vi "Teleop_old_317.vi"(10 "Match Info":T1={"Autonomous Elapsed Seconds"=0.0, "TeleOp Elapsed Seconds"=0.0, "Disabled Elapsed Seconds"=0.0, "Visited Autonomous"=FALSE, "Visited TeleOp"=FALSE, "Visited Disabled"=FALSE, "Autonomous Settings"={"Autonomous Style"=enum."Independent", "VI Refnum"=refnum}}, 11 "Call Context":T2) -> ()   [LabVIEW 2016]
doc: "This VI is called for each TeleOp packet received from the DS where the robot is not disabled. It is often used to read from the joysticks and update I/O or to update setpoints for timed control loops. It should complete and return within 20 milliseconds or it may miss DS packets."
uses:
  <vilib>/Rock Robotics/WPI/DriverStation/WPI_DriverStationDerivedRobotMode.ctl
  <vilib>/Rock Robotics/WPI/DriverStation/WPI_DriverStationMatch Info.ctl
  <vilib>/Rock Robotics/WPI/Relay/WPI_RelayValue.ctl
  <vilib>/Rock Robotics/WPI/Solenoid/WPI_SolenoidValue.ctl
  <vilib>/Rock Robotics/WPI/Utilities/WPI_GetSetVariantRefNum.vi
  <vilib>/Rock Robotics/Network Tables/NT Write Boolean Array.vi
  <vilib>/Rock Robotics/Network Tables/NT Write Numeric Array.vi
  <vilib>/Rock Robotics/Network Tables/NT Read Boolean.vi
  <vilib>/Rock Robotics/Network Tables/NT Read Number.vi
  <vilib>/Rock Robotics/WPI/Solenoid/WPI_SolenoidSetEnum.vi
panel:
  out "Feed 2":dbl(slide) scale=-1.0..1.0
  out "Feed":dbl(slide) scale=-1.0..1.0
  out "Sample Slider 0":dbl(slide) scale=0.0..5.0
  out "Sample Boolean 1":bool
  out "Sample Boolean 0":bool
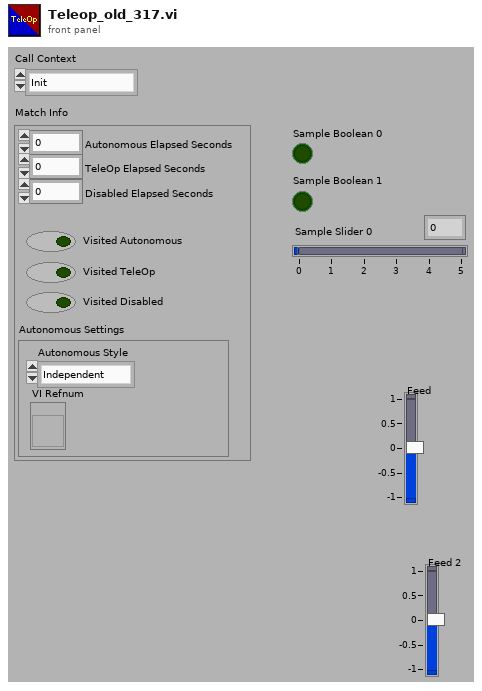
[diagram p1: front panel]
types:
  T1 = typedef "WPI_DriverStationMatch Info.ctl" = cluster{"Autonomous Elapsed Seconds":dbl, "TeleOp Elapsed Seconds":dbl, "Disabled Elapsed Seconds":dbl, "Visited Autonomous":bool, "Visited TeleOp":bool, "Visited Disabled":bool, "Autonomous Settings":cluster{"Autonomous Style":enum16{"Iterative", "Independent"}, "VI Refnum":refnum<vi>}}
  T2 = typedef "WPI_DriverStationDerivedRobotMode.ctl" = enum16{"Init", "Execute", "Stop"}
  T3 = typedef "WPI_JoystickDevRef.ctl" = cluster{"Device":T4}
  T4 = typedef "WPI_JoystickDeviceEnum.ctl" = enum16{"USB 0", "USB 1", "USB 2", "USB 3", "USB 4", "USB 5"}
  T5 = cluster{"Buttons[0]":bool, "Buttons[1]":bool, "Buttons[2]":bool, "Buttons[3]":bool, "Buttons[4]":bool, "Buttons[5]":bool, "Buttons[6]":bool, "Buttons[7]":bool, "Buttons[8]":bool, "Buttons[9]":bool, "Buttons[10]":bool}
  T6 = typedef "WPI_MotorControlDeviceRef.ctl" = cluster{"DeviceStatus":errorcluster, "Type":T7, "PWM":cluster{"PWM Channel":T8, "DeadBand":T9}, "CAN":cluster{"Device Number":u8, "SetOutput VI Ref":variant, "GetOutput VI Ref":variant, "Enable VI Ref":variant, "Disable VI Ref":variant, "Data":variant}, "Invert":bool}
  T7 = typedef "WPI_MotorControlType.ctl" = enum16{"PWM", "CAN"}
  T8 = typedef "FPGA_DIOPWMChannel.ctl" = enum8{"PWM 0", "PWM 1", "PWM 2", "PWM 3", "PWM 4", "PWM 5", "PWM 6", "PWM 7", "PWM 8", "PWM 9", "PWM MXP 0", "PWM MXP 1", "PWM MXP 2", "PWM MXP 3", "PWM MXP 4", "PWM MXP 5", "PWM MXP 6", "PWM MXP 7", "PWM MXP 8", "PWM MXP 9", "Invalid"}
  T9 = typedef "WPI_PWMDeadband.ctl" = cluster{"Name":string, "maxPositivePwm":i32, "minPositivePwm":i32, "centerPwm":i32, "maxNegativePwm":i32, "minNegativePwm":i32, "angularRange":u16}
  T10 = typedef "WPI_RelayDevRef.ctl" = cluster{"DevStatus":errorcluster, "Relay Channel":T11, "Relay Direction":T12}
  T11 = typedef "FPGA_DIORelayChannel.ctl" = enum8{"Relay 0", "Relay 1", "Relay 2", "Relay 3", "Invalid"}
  T12 = typedef "WPI_RelayDirection.ctl" = enum16{"Both directions", "Forward only", "Reverse only"}
  T13 = typedef "WPI_RobotDriveDevRef.ctl" = cluster{"DevStatus":errorcluster, "Motors[]":T6[], "Square Inputs":bool, "Max Output":dbl}
  T14 = typedef "WPI_SolenoidDevRef.ctl" = cluster{"DevStatus":errorcluster, "Pneumatics Control Module":u8, "Forward Solenoid Channel":T15, "Reverse Solenoid Channel":T15}
  T15 = typedef "WPI_SolenoidChannel.ctl" = enum8{"Solenoid 0", "Solenoid 1", "Solenoid 2", "Solenoid 3", "Solenoid 4", "Solenoid 5", "Solenoid 6", "Solenoid 7", "Invalid"}
  T16 = cluster{"Axes[0]":dbl, "Axes[1]":dbl, "Axes[2]":dbl, "Axes[3]":dbl, "Axes[4]":dbl, "Axes[5]":dbl, "Axes[6]":dbl, "Axes[7]":dbl, "Axes[8]":dbl}
  T17 = typedef "WPI_SolenoidValue.ctl" = enum16{"Off", "On", "Forward", "Reverse"}
  T18 = typedef "WPI_RelayValue.ctl" = enum16{"Off", "On", "Forward", "Reverse"}
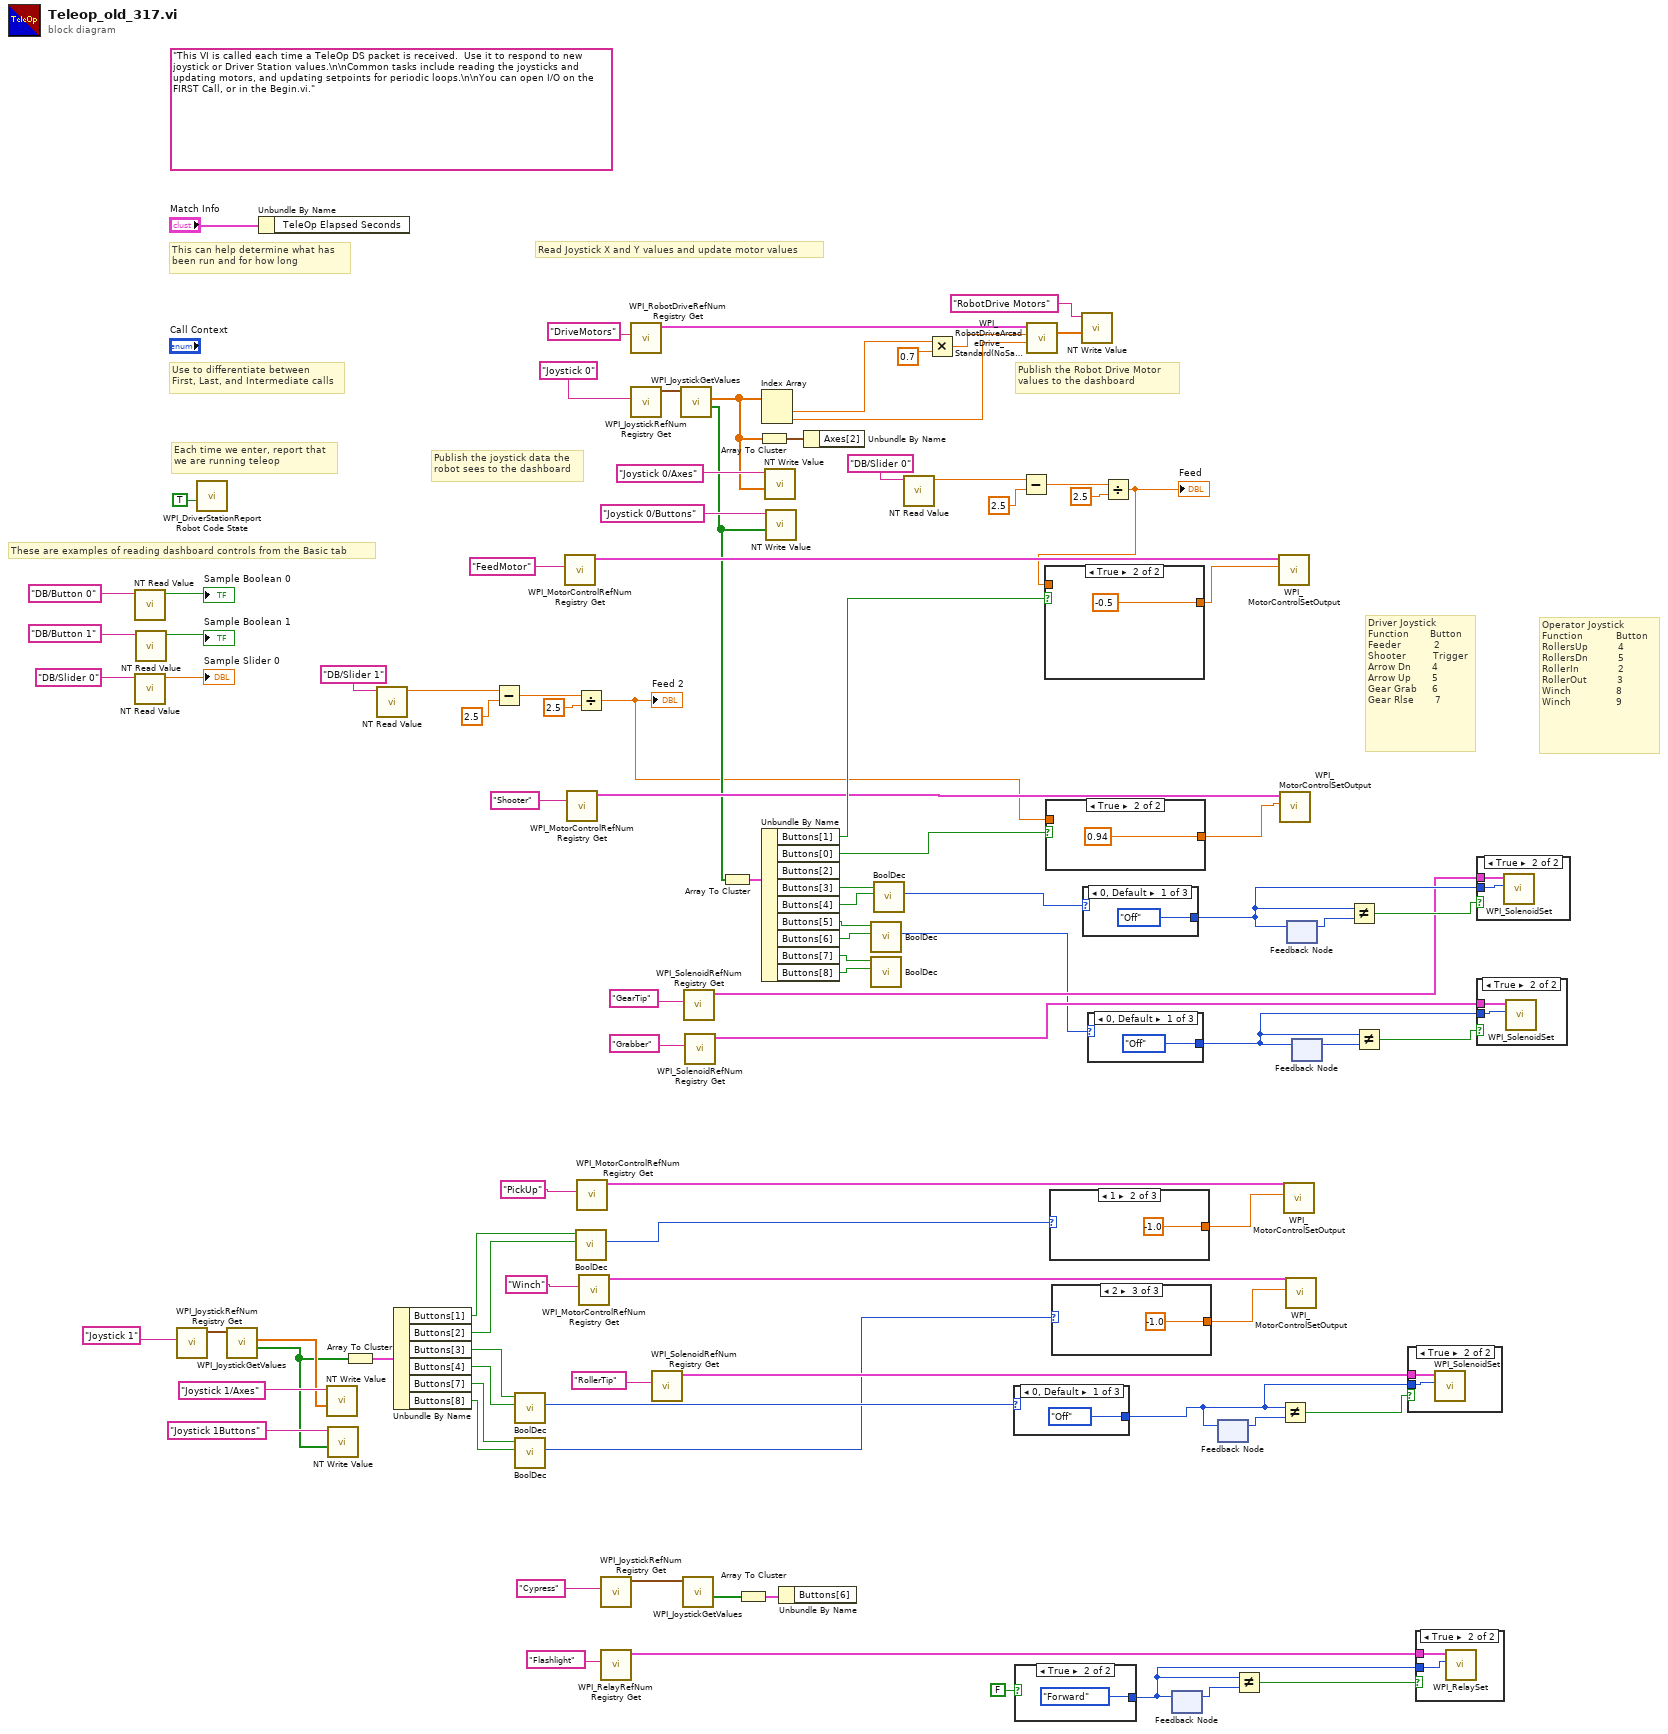
[diagram p0: block diagram]
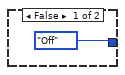
[diagram p3: hidden frame]
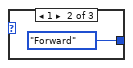
[diagram p4: hidden frame]
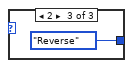
[diagram p5: hidden frame]
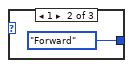
[diagram p6: hidden frame]
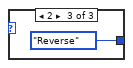
[diagram p7: hidden frame]
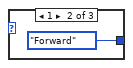
[diagram p11: hidden frame]
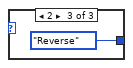
[diagram p12: hidden frame]
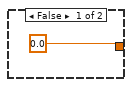
[diagram p13: hidden frame]
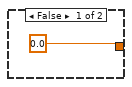
[diagram p14: hidden frame]
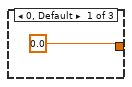
[diagram p15: hidden frame]
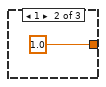
[diagram p16: hidden frame]
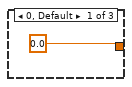
[diagram p17: hidden frame]
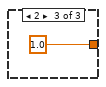
[diagram p18: hidden frame]
diagram:
  (unwired) "This VI is called each time a TeleOp DS packet is received.  Use it to respond to new joystick or Driver Station values.\n\nCommon tasks include reading the joysticks and updating motors, and updating setpoints for periodic loops.\n\nYou can open I/O on the FIRST Call, or in the Begin.vi."
  # "Operator Joystick\nFunction           Button\nRollersUp          4\nRollersDn          5\nRollerIn             2\nRollerOut          3\nWinch               8\nWinch               9"
  # "Driver Joystick\nFunction       Button\nFeeder           2\nShooter         Trigger\nArrow Dn       4\nArrow Up       5\nGear Grab     6\nGear Rlse       7"
  # "These are examples of reading dashboard controls from the Basic tab"
  # "Publish the Robot Drive Motor\nvalues to the dashboard"
  # "Publish the joystick data the\nrobot sees to the dashboard"
  # "Each time we enter, report that\nwe are running teleop"
  # "Use to differentiate between\nFirst, Last, and Intermediate calls"
  # "This can help determine what has\nbeen run and for how long"
  # "Read Joystick X and Y values and update motor values"
  n1 = call-poly <vilib>:"NT Read Value.vi"("Name"="DB/Button 0" ("refnum name")) -> ("Boolean"=→"Sample Boolean 0":bool)  [unwired: 9 in, 1 out]
  n2 = call-poly <vilib>:"NT Read Value.vi"("Name"="DB/Slider 0" ("refnum name")) -> ("Numeric"=→"Sample Slider 0":dbl)  [unwired: 9 in, 1 out]
  n3 = call-poly <vilib>:"NT Read Value.vi"("Name"="DB/Button 1" ("refnum name")) -> ("Boolean"=→"Sample Boolean 1":bool)  [unwired: 9 in, 1 out]
  n4 = call <vilib>:"WPI_JoystickRefNum Registry Get.vi"("refnum name"="Joystick 1") -> ("JoystickDevRef"=w63:T3)  [unwired: 1 in, 9 out]
  n5 = call <vilib>:"WPI_DriverStationReport Robot Code State.vi"("TeleOp"=TRUE ("Autonomous")) -> ()  [unwired: 10 in, 1 out]
  n6 = call <vilib>:"WPI_JoystickGetValues.vi"("JoystickDevRef"=w63) -> ("Buttons"=w53:bool[], "Axes"=w59:dbl[])  [unwired: 6 in, 3 out]
  n7 = Unbundle By Name("Match Info") -> ()  [unwired: 1 out]
  n8 = call-poly <vilib>:"NT Write Value.vi"("Numeric Array"=w59, "Name"="Joystick 1/Axes") -> ()  [unwired: 9 in, 1 out]
  n9 = call-poly <vilib>:"NT Write Value.vi"("Boolean Array"=w53, "Name"="Joystick 1Buttons") -> ()  [unwired: 9 in, 1 out]
  n10 = Array To Cluster(array=w53) -> (cluster=w52:T5)
  n11 = call-poly <vilib>:"NT Read Value.vi"("Name"="DB/Slider 1") -> ("Numeric"=w24:dbl)  [unwired: 9 in, 1 out]
  n12 = Unbundle By Name(w52) -> ("Buttons[1]"=w49:bool, "Buttons[2]"=w48:bool, "Buttons[3]"=w51:bool, "Buttons[4]"=w50:bool, "Buttons[7]"=w43:bool, "Buttons[8]"=w42:bool)
  n13 = Subtract(x=w24, y=2.5) -> (x-y=w22:dbl)
  n14 = call "BoolDec.vi"("Bit0"=w51, "Bit1"=w50) -> ("Out"=w7:i8)  [unwired: 8 in]
  n15 = call "BoolDec.vi"("Bit0"=w43, "Bit1"=w42) -> ("Out"=w5:i8)  [unwired: 8 in]
  n16 = call <vilib>:"WPI_MotorControlRefNum Registry Get.vi"("refnum name"="FeedMotor") -> ("MotorControlDevRef"=w66:T6)  [unwired: 9 in, 1 out]
  n17 = call <vilib>:"WPI_MotorControlRefNum Registry Get.vi"("refnum name"="Shooter") -> ("MotorControlDevRef"=w67:T6)  [unwired: 9 in, 1 out]
  n18 = Divide(x=w22, y=2.5) -> (x/y=w14:dbl)
  "Feed 2" <- w14
  n19 = call "BoolDec.vi"("Bit0"=w49, "Bit1"=w48) -> ("Out"=w6:i8)  [unwired: 8 in]
  n20 = call <vilib>:"WPI_MotorControlRefNum Registry Get.vi"("refnum name"="PickUp") -> ("MotorControlDevRef"=w78:T6)  [unwired: 9 in, 1 out]
  n21 = call <vilib>:"WPI_MotorControlRefNum Registry Get.vi"("refnum name"="Winch") -> ("MotorControlDevRef"=w71:T6)  [unwired: 9 in, 1 out]
  n22 = call <vilib>:"WPI_JoystickRefNum Registry Get.vi"("refnum name"="Cypress") -> ("JoystickDevRef"=w3:T3)  [unwired: 9 in, 1 out]
  n23 = call <vilib>:"WPI_RelayRefNum Registry Get.vi"("refnum name"="Flashlight") -> ("RelayDevRef"=w19:T10)  [unwired: 9 in, 1 out]
  n24 = call <vilib>:"WPI_RobotDriveRefNum Registry Get.vi"("refnum name"="DriveMotors") -> ("RobotDriveDevRef"=w97:T13)  [unwired: 1 in, 9 out]
  n25 = call <vilib>:"WPI_JoystickRefNum Registry Get.vi"("refnum name"="Joystick 0") -> ("JoystickDevRef"=w95:T3)  [unwired: 1 in, 9 out]
  n26 = call <vilib>:"WPI_SolenoidRefNum Registry Get.vi"("refnum name"="RollerTip") -> ("SolenoidDevRef"=w54:T14)  [unwired: 9 in, 1 out]
  n27 = call <vilib>:"WPI_JoystickGetValues.vi"("JoystickDevRef"=w95) -> ("Buttons"=w58:bool[], "Axes"=w80:dbl[])  [unwired: 6 in, 3 out]
  n28 = call <vilib>:"WPI_JoystickGetValues.vi"("JoystickDevRef"=w3) -> ("Buttons"=w2:bool[])  [unwired: 6 in, 4 out]
  n29 = call <vilib>:"WPI_SolenoidRefNum Registry Get.vi"("refnum name"="GearTip") -> ("SolenoidDevRef"=w10:T14)  [unwired: 9 in, 1 out]
  n30 = call <vilib>:"WPI_SolenoidRefNum Registry Get.vi"("refnum name"="Grabber") -> ("SolenoidDevRef"=w9:T14)  [unwired: 9 in, 1 out]
  n31 = Array To Cluster(array=w58) -> (cluster=w81:T5)
  n32 = Array To Cluster(array=w2) -> (cluster=w1:T5)
  n33 = Array To Cluster(array=w80) -> (cluster=w79:T16)
  n34 = Index Array(array=w80) -> (element #1=w34:dbl, element #2=w93:dbl)  [unwired: 2 in]
  n35 = Unbundle By Name(w81) -> ("Buttons[1]"=w68:bool, "Buttons[0]"=w69:bool, "Buttons[3]"=w13:bool, "Buttons[4]"=w12:bool, "Buttons[5]"=w76:bool, "Buttons[6]"=w75:bool, "Buttons[7]"=w74:bool, "Buttons[8]"=w73:bool)  [unwired: 1 out]
  n36 = call-poly <vilib>:"NT Write Value.vi"("Numeric Array"=w80, "Name"="Joystick 0/Axes") -> ()  [unwired: 9 in, 1 out]
  n37 = call-poly <vilib>:"NT Write Value.vi"("Boolean Array"=w58, "Name"="Joystick 0/Buttons") -> ()  [unwired: 9 in, 1 out]
  n38 = Unbundle By Name(w1) -> ()  [unwired: 1 out]
  n39 = Unbundle By Name(w79) -> ()  [unwired: 1 out]
  n40 = call "BoolDec.vi"("Bit0"=w76, "Bit1"=w75) -> ("Out"=w8:i8)  [unwired: 8 in]
  n41 = call "BoolDec.vi"("Bit0"=w74, "Bit1"=w73) -> ()  [unwired: 8 in, 1 out]
  n42 = call "BoolDec.vi"("Bit0"=w13, "Bit1"=w12) -> ("Out"=w11:i8)  [unwired: 8 in]
  n43 = call-poly <vilib>:"NT Read Value.vi"("Name"="DB/Slider 0") -> ("Numeric"=w30:dbl)  [unwired: 9 in, 1 out]
  n44 = Multiply(x=w34, y=0.7) -> (x*y=w32:dbl)
  n45 = case shown="0, Default" w7 {
    tunnel: [WPI_SolenoidValue."Off" ("Value") WPI_SolenoidValue."Forward" ("Value") WPI_SolenoidValue."Reverse" ("Value")] -> w37
    frame 0, Default {
    }
    frame 1 {
    }
    frame 2 {
    }
  }
  n46 = case shown="True" FALSE {
    tunnel: [WPI_RelayValue."Off" ("RelayValue") WPI_RelayValue."Forward" ("RelayValue")] -> w15
    frame False {
    }
    frame True {
    }
  }
  n47 = Subtract(x=w30, y=2.5) -> (x-y=w28:dbl)
  n48 = call <vilib>:"WPI_RobotDriveArcadeDrive_Standard(NoSaturation).vi"("Y axis value"=w93, "X axis value"=w32, "RobotDriveDevRef"=w97) -> ("Motor Values"=w84:dbl[])  [unwired: 1 in, 7 out]
  n49 = case shown="True" w69 {
    tunnel: [0.0 ("Output") 0.94] -> w35
    tunnel: w14 -> [_ _]
    frame False {
    }
    frame True {
    }
  }
  n50 = case shown="1" w6 {
    tunnel: [0.0 ("Output") -1.0 1.0] -> w77
    frame 0, Default {
    }
    frame 1 {
    }
    frame 2 {
    }
  }
  n51 = case shown="2" w5 {
    tunnel: [0.0 ("Output") 1.0 -1.0] -> w72
    frame 0, Default {
    }
    frame 1 {
    }
    frame 2 {
    }
  }
  n52 = call-poly <vilib>:"NT Write Value.vi"("Numeric Array"=w84, "Name"="RobotDrive Motors") -> ()  [unwired: 9 in, 1 out]
  n53 = case shown="0, Default" w11 {
    tunnel: [WPI_SolenoidValue."Off" ("Value") WPI_SolenoidValue."Forward" ("Value") WPI_SolenoidValue."Reverse" ("Value")] -> w38
    frame 0, Default {
    }
    frame 1 {
    }
    frame 2 {
    }
  }
  n54 = case shown="0, Default" w8 {
    tunnel: [WPI_SolenoidValue."Off" ("Value") WPI_SolenoidValue."Forward" ("Value") WPI_SolenoidValue."Reverse" ("Value")] -> w39
    frame 0, Default {
    }
    frame 1 {
    }
    frame 2 {
    }
  }
  n55 = Divide(x=w28, y=2.5) -> (x/y=w26:dbl)
  "Feed" <- w26
  n56 = case shown="True" w68 {
    tunnel: [0.0 ("Output") -0.5] -> w36
    tunnel: w26 -> [_ _]
    frame False {
    }
    frame True {
    }
  }
  n57 = feedback #1() -> (w18:T18)  [unwired: 1 in]
  n58 = feedback-in #1(w15) -> ()
  n59 = feedback #2() -> (w44:T17)  [unwired: 1 in]
  n60 = feedback-in #2(w37) -> ()
  n61 = Not Equal?(x=w15, y=w18) -> (x != y?=w17:bool)
  n62 = call <vilib>:"WPI_MotorControlSetOutput.vi"("Output"=w36, "MotorControlDevRef"=w66) -> ()  [unwired: 7 in, 3 out]
  n63 = call <vilib>:"WPI_MotorControlSetOutput.vi"("Output"=w35, "MotorControlDevRef"=w67) -> ()  [unwired: 7 in, 3 out]
  n64 = Not Equal?(x=w37, y=w44) -> (x != y?=w40:bool)
  n65 = call <vilib>:"WPI_MotorControlSetOutput.vi"("Output"=w77, "MotorControlDevRef"=w78) -> ()  [unwired: 7 in, 3 out]
  n66 = call <vilib>:"WPI_MotorControlSetOutput.vi"("Output"=w72, "MotorControlDevRef"=w71) -> ()  [unwired: 7 in, 3 out]
  n67 = feedback #3() -> (w45:T17)  [unwired: 1 in]
  n68 = feedback-in #3(w38) -> ()
  n69 = feedback-in #4(w39) -> ()
  n70 = feedback #4() -> (w46:T17)  [unwired: 1 in]
  n71 = Not Equal?(x=w38, y=w45) -> (x != y?=w41:bool)
  n72 = Not Equal?(x=w39, y=w46) -> (x != y?=w47:bool)
  n73 = case shown="True" w40 {
    tunnel: w54 -> [_ w122]
    tunnel: w37 -> [_ w121]
    frame False {
    }
    frame True {
      n74 = call-poly <vilib>:"WPI_SolenoidSet.vi"("Value"=w121, "SolenoidDevRef"=w122) -> ()  [unwired: 8 in, 2 out]
    }
  }
  n75 = case shown="True" w17 {
    tunnel: w19 -> [_ w124]
    tunnel: w15 -> [_ w123]
    frame False {
    }
    frame True {
      n76 = call <vilib>:"WPI_RelaySet.vi"("RelayValue"=w123, "RelayDevRef"=w124) -> ()  [unwired: 8 in, 2 out]
    }
  }
  n77 = case shown="True" w41 {
    tunnel: w10 -> [_ w126]
    tunnel: w38 -> [_ w125]
    frame False {
    }
    frame True {
      n78 = call-poly <vilib>:"WPI_SolenoidSet.vi"("Value"=w125, "SolenoidDevRef"=w126) -> ()  [unwired: 8 in, 2 out]
    }
  }
  n79 = case shown="True" w47 {
    tunnel: w9 -> [_ w128]
    tunnel: w39 -> [_ w127]
    frame False {
    }
    frame True {
      n80 = call-poly <vilib>:"WPI_SolenoidSet.vi"("Value"=w127, "SolenoidDevRef"=w128) -> ()  [unwired: 8 in, 2 out]
    }
  }
